vi "Capture.vi"(0 "Commands array":string[][](array[string])=[["Group20.825", "Group20.671", "Group20.814", "Group30.121"], ["Group2-0.528", "Group2-1.243", "Group2-0.539", "Group30.121"], ["Group20.374", "Group21.573", "Group20.363", "Group30.121"], ["Group2-0.242", "Group2-1.815", "Group2-0.253", "Group30.121"], ["Group20.165", "Group21.991", "Group20.154", "Group30.121"], ["Group2-0.077", "Group2-2.145", "Group2-0.088", "Group30.121"], ["Group20.044", "Group22.233", "Group20.033", "Group30.121"], ["Group2-2.310", "WT10", "WT10", "Group30.121"], ["Group22.310", "WT10", "WT10", "Group30.121"], ["Group2-2.310", "WT10", "WT10", "Group30.121"], ["Group22.310", "WT10", "WT10", "Group30.121"], ["Group2-2.310", "WT10", "WT10", "Group30.121"], ["Group22.310", "WT10", "WT10", "Group30.121"], ["Group2-0.011", "Group2-2.277", "Group2-0.022", "Group30.121"], ["Group20.066", "Group22.189", "Group20.055", "Group30.121"], ["Group2-0.121", "Group2-2.057", "Group2-0.132", "Group30.121"], ["Group20.209", "Group21.903", "Group20.198", "Group30.121"], ["Group2-0.297", "Group2-1.705", "Group2-0.308", "Group30.121"], ["Group20.451", "Group21.419", "Group20.440", "Group30.121"], ["Group2-0.660", "Group2-0.979", "Group2-0.671", "Group30.121"]], 1 "XPS_Address":string="192.168.254.254", 2 "VISA resource name":refnum<visa-resource-name>, 3 "laser array index":i32, 4 "Process time":dbl format="%#_13g", 5 "Axis Speed":dbl=1.0 format="%#_13g", 6 "Laser on/off array":bool[][](array[boolean])=[[FALSE, TRUE, FALSE, FALSE], [FALSE, TRUE, FALSE, FALSE], [FALSE, TRUE, FALSE, FALSE], [FALSE, TRUE, FALSE, FALSE], [FALSE, TRUE, FALSE, FALSE], [FALSE, TRUE, FALSE, FALSE], [FALSE, TRUE, FALSE, FALSE], [TRUE, FALSE, FALSE, FALSE], [TRUE, FALSE, FALSE, FALSE], [TRUE, FALSE, FALSE, FALSE], [TRUE, FALSE, FALSE, FALSE], [TRUE, FALSE, FALSE, FALSE], [TRUE, FALSE, FALSE, FALSE], [FALSE, TRUE, FALSE, FALSE], [FALSE, TRUE, FALSE, FALSE], [FALSE, TRUE, FALSE, FALSE], [FALSE, TRUE, FALSE, FALSE], [FALSE, TRUE, FALSE, FALSE], [FALSE, TRUE, FALSE, FALSE], [FALSE, TRUE, FALSE, FALSE]], 7 "stop":bool, 8 "delay before read (ms)":u32=500, 11 "Axis Initial Parameters":T1={"Velocity (units/seconds)"=1.0, "Acceleration (units/seconds²)"=20.0, "Minimum Jerk Time (seconds)"=0.005, "Maximum Jerk Time (seconds)"=0.009} {"Maximum Jerk Time (seconds)" format="%.6e"; "Minimum Jerk Time (seconds)" format="%.6e"; "Acceleration (units/seconds²)" format="%.6e"; "Velocity (units/seconds)" format="%.6e"}, 13 "ROI Area \n(mm2)":dbl=4.035870075999999, 14 "Axis 2":string="Group3", 15 "Axis 1":string="Group2", 17 "OPO on?":bool, 19 "Acceleration (units/seconds²)":dbl=20.0) -> (10 "Elapsed time":dbl, 16 "XPS error out":errorcluster, 18 "Error out":errorcluster)   [LabVIEW 2016]
uses:
  case selector.ctl
panel:
  out "Capture Log":string
  out "Axis 1 position":dbl format="%.10f"
  out "Axis 2 position":dbl format="%.10f"
  out "Initial time":timestamp
  in  "Active Positioner":string
  out "Current Line":i32
  out "1D Laser Array":bool[](array[boolean])=[FALSE, TRUE, FALSE, FALSE, FALSE, TRUE, FALSE, FALSE, FALSE, TRUE, FALSE, FALSE, FALSE, TRUE, FALSE, FALSE, FALSE, TRUE, FALSE, FALSE, FALSE, TRUE, FALSE, FALSE, FALSE, TRUE, FALSE, FALSE, TRUE, FALSE, FALSE, FALSE, TRUE, FALSE, FALSE, FALSE, TRUE, FALSE, FALSE, FALSE, TRUE, FALSE, FALSE, FALSE, TRUE, FALSE, FALSE, FALSE, TRUE, FALSE, FALSE, FALSE, FALSE, TRUE, FALSE, FALSE, FALSE, TRUE, FALSE, FALSE, FALSE, TRUE, FALSE, FALSE, FALSE, TRUE, FALSE, FALSE, FALSE, TRUE, FALSE, FALSE, FALSE, TRUE, FALSE, FALSE, FALSE, TRUE, FALSE, FALSE]
  out "1D command array":string[](array[string])=["Group20.825", "Group20.671", "Group20.814", "Group30.121", "Group2-0.528", "Group2-1.243", "Group2-0.539", "Group30.121", "Group20.374", "Group21.573", "Group20.363", "Group30.121", "Group2-0.242", "Group2-1.815", "Group2-0.253", "Group30.121", "Group20.165", "Group21.991", "Group20.154", "Group30.121", "Group2-0.077", "Group2-2.145", "Group2-0.088", "Group30.121", "Group20.044", "Group22.233", "Group20.033", "Group30.121", "Group2-2.310", "WT10", "WT10", "Group30.121", "Group22.310", "WT10", "WT10", "Group30.121", "Group2-2.310", "WT10", "WT10", "Group30.121", "Group22.310", "WT10", "WT10", "Group30.121", "Group2-2.310", "WT10", "WT10", "Group30.121", "Group22.310", "WT10", "WT10", "Group30.121", "Group2-0.011", "Group2-2.277", "Group2-0.022", "Group30.121", "Group20.066", "Group22.189", "Group20.055", "Group30.121", "Group2-0.121", "Group2-2.057", "Group2-0.132", "Group30.121", "Group20.209", "Group21.903", "Group20.198", "Group30.121", "Group2-0.297", "Group2-1.705", "Group2-0.308", "Group30.121", "Group20.451", "Group21.419", "Group20.440", "Group30.121", "Group2-0.660", "Group2-0.979", "Group2-0.671", "Group30.121"]
  out "Current Command":string
  out "Current laser element":bool
  out "Total lines":i32=80
  in  "Active Axis":string
  out "Laser on/off":bool
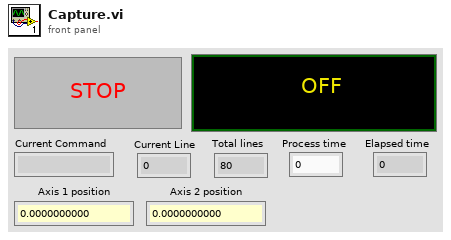
[diagram p1: front panel]
types:
  T1 = cluster{"Velocity (units/seconds)":dbl, "Acceleration (units/seconds²)":dbl, "Minimum Jerk Time (seconds)":dbl, "Maximum Jerk Time (seconds)":dbl}
  T2 = typedef "case selector.ctl" = enum16{"Initialize", "Element selection", "Laser", "Velocities", "Command", "Wait", "Exit"}
  T3 = enum16{"open", "replace", "create", "open or create", "replace or create", "replace or create with confirmation"}
  T4 = cluster{"connection TCP":refnum<k5>, "LogTo File":bool, "Log File refnum":refnum<file>, "no error if error log":bool}
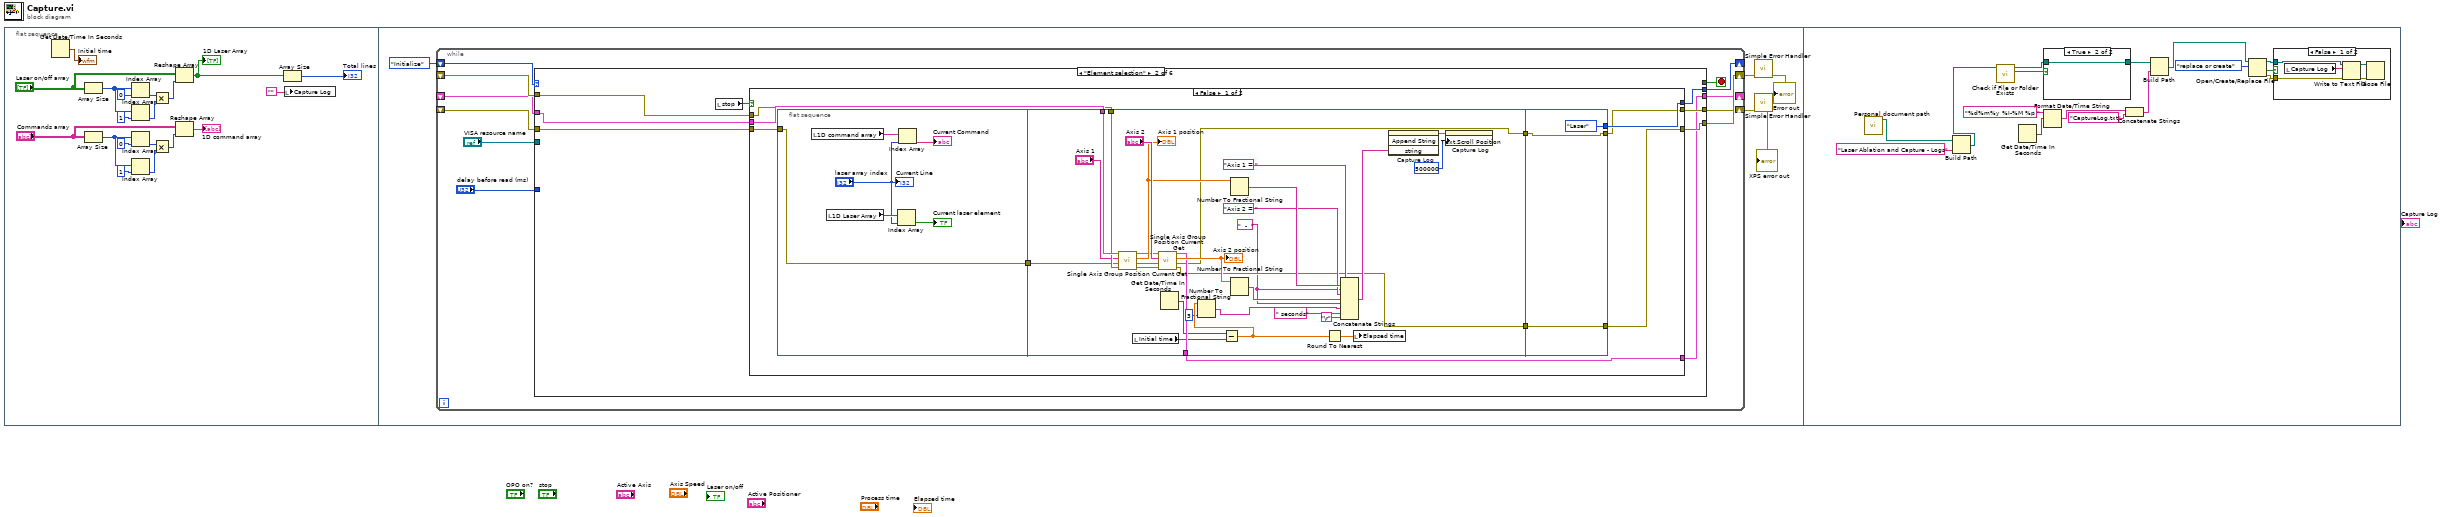
[diagram p0: block diagram]
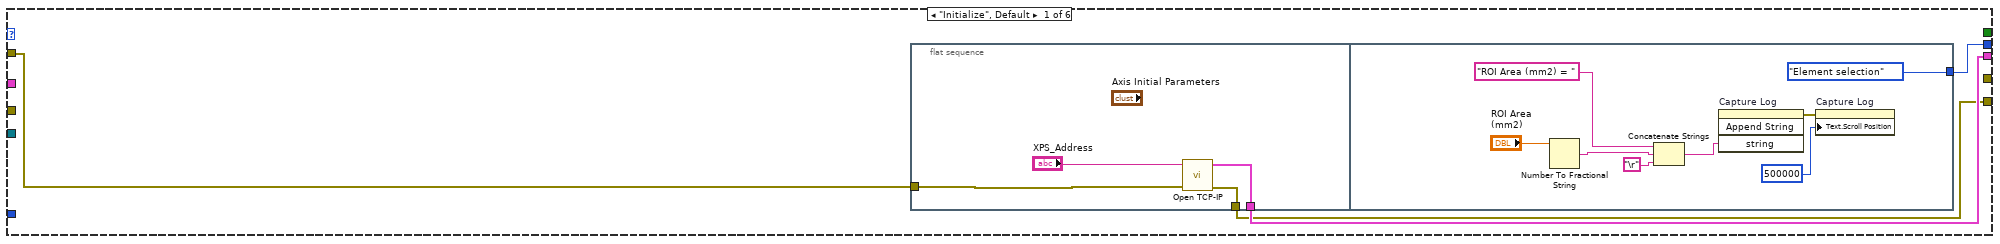
[diagram p2: hidden frame]
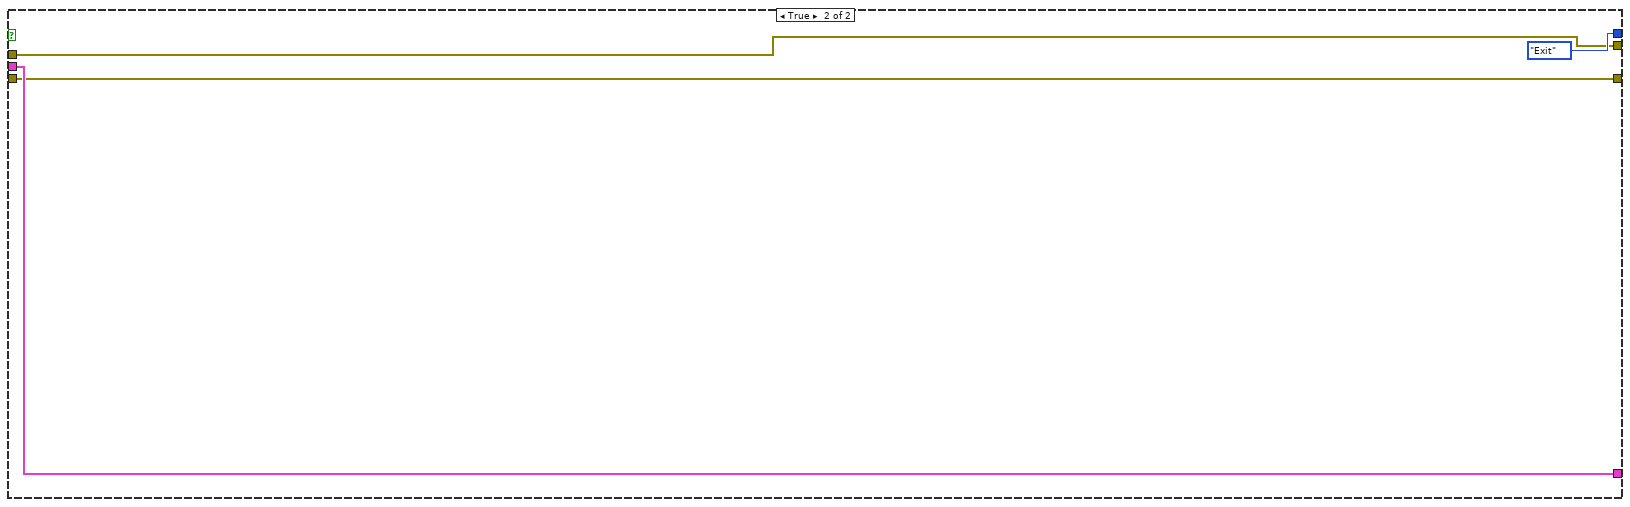
[diagram p3: hidden frame]
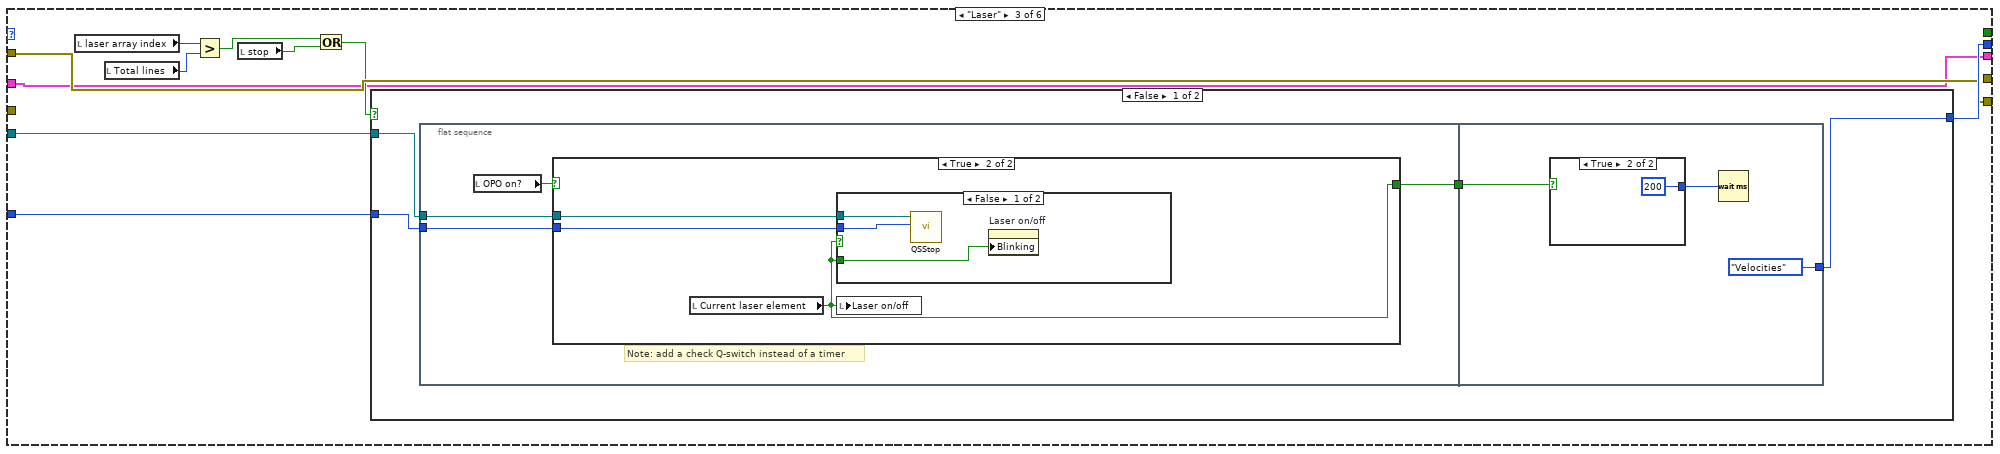
[diagram p4: hidden frame]
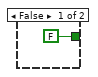
[diagram p5: hidden frame]
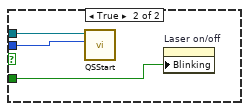
[diagram p6: hidden frame]
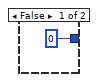
[diagram p7: hidden frame]
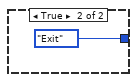
[diagram p8: hidden frame]
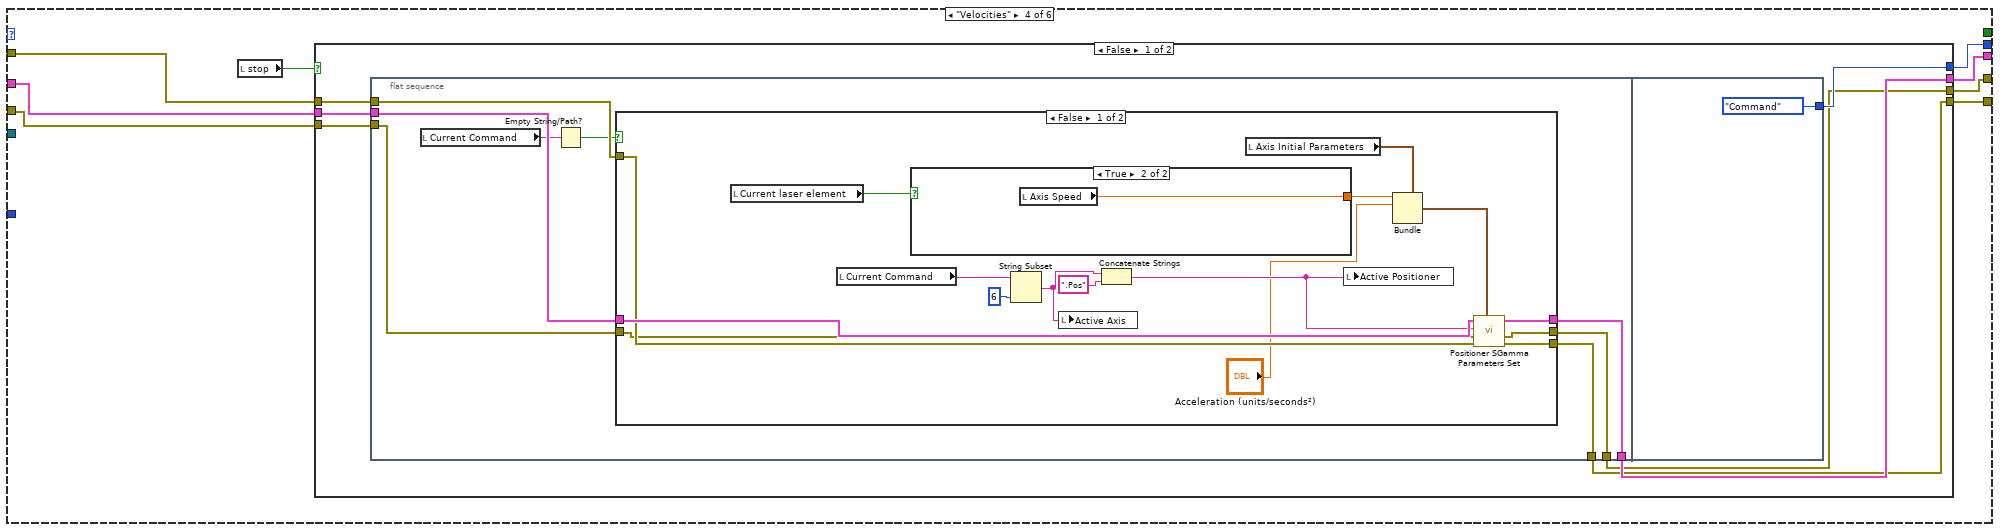
[diagram p9: hidden frame]
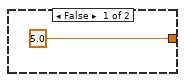
[diagram p10: hidden frame]
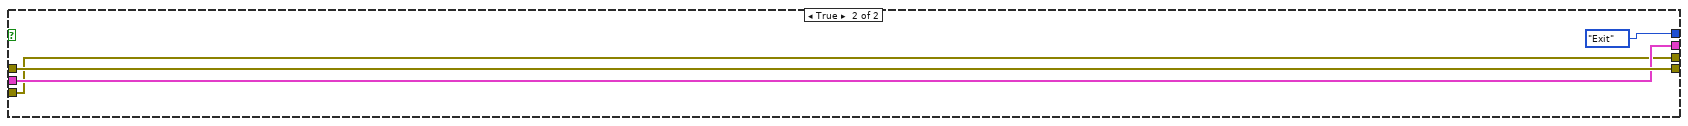
[diagram p12: hidden frame]
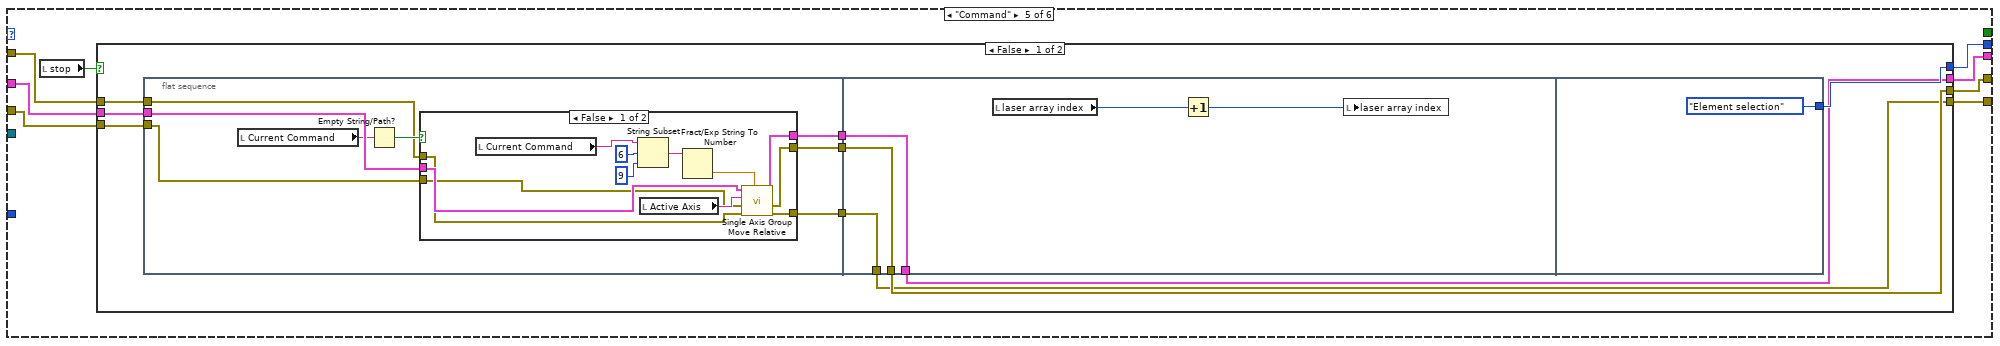
[diagram p13: hidden frame]
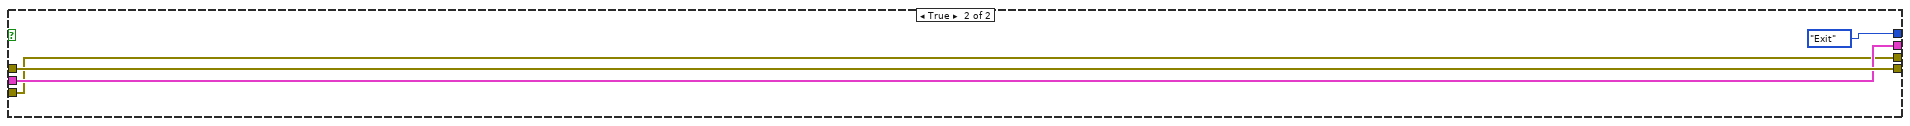
[diagram p15: hidden frame]
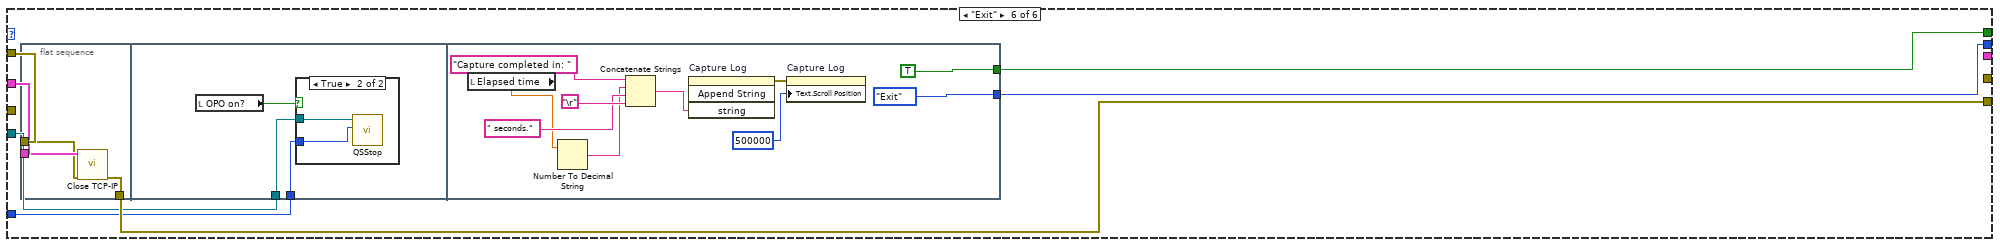
[diagram p16: hidden frame]
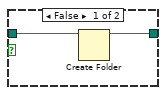
[diagram p18: hidden frame]
diagram:
  n1 = flat-sequence {
    frame #0 {
      n2 = Get Date/Time In Seconds() -> (seconds since 1Jan1904=→"Initial time":timestamp)
      n3 = Array Size(array="Commands array") -> (size(s)=w3:i32[])
      n4 = Array Size(array="Laser on/off array") -> (size(s)=w11:i32[])
      n5 = Index Array(array=w11, index=0) -> (element=w14:i32)
      n6 = Index Array(array=w11, index=1) -> (element=w15:i32)
      n7 = Index Array(array=w3, index=0) -> (element=w6:i32)
      n8 = Index Array(array=w3, index=1) -> (element=w7:i32)
      n9 = Multiply(x=w14, y=w15) -> (x*y=w16:i32)
      n10 = Multiply(x=w6, y=w7) -> (x*y=w8:i32)
      n11 = Reshape Array("Laser on/off array", w16) -> (w19:bool[])
      "1D Laser Array" <- w19
      n12 = Reshape Array("Commands array", w8) -> (→"1D command array":string[])
      n13 = Array Size(array=w19) -> (size(s)=→"Total lines":i32)
      n14 = local write "Capture Log"("") -> ()
    }
    frame #1 {
      n15 = while {
        shift-right: [w32] -> _
        shift-left: case_selector."Initialize" -> [w33]
        shift-right: [w30] -> w20
        shift-left: _ -> [w31]
        shift-right: [w29] -> _
        shift-left: _ -> [w28]
        shift-right: [w27] -> w21
        shift-left: _ -> [w26]
        stop <- w25 stop-if-true
        n16 = case shown="\"Element selection\"" w33 {
          tunnel: [w37 w57 w119 w151 w200 w247] -> w32
          tunnel: w31 -> [w36 w54 w118 w149 w198 w248]
          tunnel: [w34 w51 w118 w148 w197 w246] -> w30
          tunnel: [w35 w50 w112 w146 w195 _] -> w29
          tunnel: w28 -> [_ w55 w112 w147 w196 w245]
          tunnel: [_ w52 _ w145 w193 _] -> w27
          tunnel: w26 -> [_ w53 _ w144 w194 _]
          tunnel: [_ _ _ _ _ w244] -> w25
          tunnel: "VISA resource name" -> [_ _ w111 _ _ w242]
          tunnel: "delay before read (ms)" -> [_ _ w110 _ _ w243]
          frame "Initialize", Default {
            n17 = flat-sequence {
              tunnel: w36 -> [w40]
              tunnel: [w39] -> w35
              tunnel: [w38] -> w34
              tunnel: [case_selector."Element selection"] -> w37
              frame #0 {
                n18 = call <userlib>:"Open TCP-IP.vi"("error in (no error)"=w40, "IP address"="XPS_Address") -> ("error out"=w38:errorcluster, "Connection ID"=w39:T4)  [unwired: 7 in, 1 out]
              }
              frame #1 {
                n19 = Number To Fractional String(number="ROI Area \n(mm2)") -> (F-format string=w45:string)  [unwired: 3 in]
                n20 = Concatenate Strings("ROI Area (mm2) = " ("string"), w45, "\r") -> (w43:string)
                n21 = invoke on="Capture Log" class="Str" method="Append String"("string"=w43) -> (error out=w47:errorcluster)  [unwired: 3 in, 3 out]
                n22 = property on="Capture Log" class="Str"(error in=w47, "Text.Scroll Position"=u32 500000) -> ()  [unwired: 1 in, 2 out]
              }
            }
          }
          frame "Element selection" {
            n23 = local read "stop"() -> (w56:bool)
            n24 = case shown="False" w56 {
              tunnel: [w66 case_selector."Exit"] -> w57
              tunnel: w55 -> [w67 w108]
              tunnel: w54 -> [w60 w107]
              tunnel: w53 -> [w59 w106]
              tunnel: [w61 w107] -> w52
              tunnel: [w63 w106] -> w51
              tunnel: [w65 w108] -> w50
              frame False {
                n25 = flat-sequence {
                  tunnel: w59 -> [w68]
                  tunnel: [w68] -> w58
                  tunnel: w67 -> [w95]
                  tunnel: w60 -> [w93]
                  tunnel: [w86] -> w65
                  tunnel: [w85] -> w64
                  tunnel: [w84] -> w62
                  tunnel: w58 -> [w83]
                  tunnel: [case_selector."Laser"] -> w66
                  tunnel: w64 -> [w104]
                  tunnel: [w104] -> w63
                  tunnel: w62 -> [w103]
                  tunnel: [w103] -> w61
                  frame #0 {
                    n26 = local read "1D command array"() -> (w71:string[])
                    n27 = local read "1D Laser Array"() -> (w70:bool[])
                    n28 = Index Array(array=w70, index="laser array index") -> (element=→"Current laser element":bool)
                    n29 = Index Array(array=w71, index="laser array index") -> (element=→"Current Command":string)
                    "Current Line" <- "laser array index"
                  }
                  frame #1 {
                    w82 = "  -  " ("string")
                    n30 = call <userlib>:"Single Axis Group Position Current Get.vi"("error in (no error)"=w93, "XPS error in (no error)"=w83, "SingleAxis Group  Name (250 c max)"="Axis 1", "connection ID in"=w95) -> ("error out"=w87:errorcluster, "XPS error out"=w88:errorcluster, "Current Position (units)"=w92:dbl, "connection ID out"=w89:T4)  [unwired: 4 in]
                    "Axis 1 position" <- w92
                    n31 = local read "Initial time"() -> (w79:timestamp)
                    n32 = call <userlib>:"Single Axis Group Position Current Get.vi"("error in (no error)"=w87, "XPS error in (no error)"=w88, "SingleAxis Group  Name (250 c max)"="Axis 2", "connection ID in"=w89) -> ("error out"=w85:errorcluster, "XPS error out"=w84:errorcluster, "Current Position (units)"=w91:dbl, "connection ID out"=w86:T4)  [unwired: 4 in]
                    "Axis 2 position" <- w91
                    n33 = Get Date/Time In Seconds() -> (seconds since 1Jan1904=w80:timestamp)
                    n34 = Subtract(x=w80, y=w79) -> (x-y=w75:dbl)
                    n35 = Number To Fractional String(number=w75, precision (6)=i16 3) -> (F-format string=w78:string)  [unwired: 2 in]
                    n36 = Number To Fractional String(number=w92) -> (F-format string=w101:string)  [unwired: 3 in]
                    n37 = Number To Fractional String(number=w91) -> (F-format string=w100:string)  [unwired: 3 in]
                    n38 = Round To Nearest(number=w75) -> (nearest integer value=w81:dbl)
                    n39 = Concatenate Strings("Axis 1 = " ("string"), w101, w82, "Axis 2 = " ("string"), w100, w82, w78, " seconds" ("milliseconds"), "\r") -> (w98:string)
                    n40 = local write "Elapsed time"(w81) -> ()
                    n41 = invoke on="Capture Log" class="Str" method="Append String"("string"=w98) -> (error out=w97:errorcluster)  [unwired: 3 in, 3 out]
                    n42 = property on="Capture Log" class="Str"(error in=w97, "Text.Scroll Position"=u32 500000) -> ()  [unwired: 1 in, 2 out]
                  }
                  frame #2 {
                  }
                }
              }
              frame True {
              }
            }
          }
          frame "Laser" {
            n43 = local read "laser array index"() -> (w116:i32)
            n44 = local read "Total lines"() -> (w117:i32)
            n45 = Greater?(x=w116, y=w117) -> (0:w114:bool)
            n46 = local read "stop"() -> (w115:bool)
            n47 = Or(x=w114, y=w115) -> (x .or. y?=w113:bool)
            n48 = case shown="False" w113 {
              tunnel: [w123 case_selector."Exit"] -> w119
              tunnel: w111 -> [w121 _]
              tunnel: w110 -> [w120 _]
              frame False {
                n49 = flat-sequence {
                  tunnel: [w126] -> w122
                  tunnel: w121 -> [w125]
                  tunnel: w120 -> [w124]
                  tunnel: [case_selector."Velocities"] -> w123
                  tunnel: w122 -> [w139]
                  frame #0 {
                    # "Note: add a check Q-switch instead of a timer"
                    n50 = local read "OPO on?"() -> (w127:bool)
                    n51 = case shown="True" w127 {
                      tunnel: [FALSE ("Current laser element") w131] -> w126
                      tunnel: w125 -> [_ w130]
                      tunnel: w124 -> [_ w129]
                      frame False {
                      }
                      frame True {
                        n52 = local read "Current laser element"() -> (w131:bool)
                        n53 = case shown="False" w131 {
                          tunnel: w131 -> [w134 w137]
                          tunnel: w130 -> [w133 w136]
                          tunnel: w129 -> [w132 w135]
                          frame False {
                            n54 = call "QSStop.vi"("delay before read (ms)"=w132, "VISA resource name"=w133) -> ()  [unwired: 6 in, 4 out]
                            n55 = property on="Laser on/off" class="Bool (strict)"("Blinking"=w134) -> ()  [unwired: 2 in, 2 out]
                          }
                          frame True {
                            n56 = call "QSStart.vi"("delay before read (ms)"=w135, "VISA resource name"=w136) -> ()  [unwired: 6 in, 4 out]
                            n57 = property on="Laser on/off" class="Bool (strict)"("Blinking"=w137) -> ()  [unwired: 2 in, 2 out]
                          }
                        }
                        n58 = local write "Laser on/off"(w131) -> ()
                      }
                    }
                  }
                  frame #1 {
                    n59 = case shown="True" w139 {
                      tunnel: [u32 0 ("milliseconds to wait") u32 200 ("milliseconds to wait")] -> w138
                      frame False {
                      }
                      frame True {
                      }
                    }
                    n60 = Wait (ms)(milliseconds to wait=w138) -> ()  [unwired: 1 out]
                  }
                }
              }
              frame True {
              }
            }
          }
          frame "Velocities" {
            n61 = local read "stop"() -> (w150:bool)
            n62 = case shown="False" w150 {
              tunnel: [w158 case_selector."Exit"] -> w151
              tunnel: w149 -> [w157 w191]
              tunnel: [w154 w191] -> w148
              tunnel: w147 -> [w156 w190]
              tunnel: [w155 w190] -> w146
              tunnel: [w153 w189] -> w145
              tunnel: w144 -> [w152 w189]
              frame False {
                n63 = flat-sequence {
                  tunnel: w157 -> [w164]
                  tunnel: w156 -> [w166]
                  tunnel: [w165] -> w155
                  tunnel: [w163] -> w154
                  tunnel: [w162] -> w153
                  tunnel: w152 -> [w161]
                  tunnel: [case_selector."Command"] -> w158
                  frame #0 {
                    n64 = local read "Current Command"() -> (w160:string)
                    n65 = Empty String/Path?(string/path=w160) -> (empty?=w159:bool)
                    n66 = case shown="False" w159 {
                      tunnel: w166 -> [w179 w185]
                      tunnel: [w178 w185] -> w165
                      tunnel: w164 -> [w177 w186]
                      tunnel: [w176 w186] -> w163
                      tunnel: [w171 w187] -> w162
                      tunnel: w161 -> [w170 w187]
                      frame False {
                        n67 = local read "Current laser element"() -> (w182:bool)
                        n68 = local read "Current Command"() -> (w180:string)
                        n69 = case shown="True" w182 {
                          tunnel: [5.0 w184] -> w175
                          frame False {
                          }
                          frame True {
                            n70 = local read "Axis Speed"() -> (w184:dbl)
                          }
                        }
                        n71 = String Subset(string=w180, length (rest)=6 ("length (rest)")) -> (substring=w169:string)  [unwired: 1 in]
                        n72 = local write "Active Axis"(w169) -> ()
                        n73 = Concatenate Strings(w169, ".Pos" ("string")) -> (w168:string)
                        n74 = local read "Axis Initial Parameters"() -> (w173:T1)
                        n75 = local write "Active Positioner"(w168) -> ()
                        n76 = Bundle(cluster=w173, "Velocity (units/seconds)"=w175, "Acceleration (units/seconds²)"="Acceleration (units/seconds²)") -> (w174:T1)  [unwired: 2 in]
                        n77 = call <userlib>:"Positioner SGamma Parameters Set.vi"("SGamma Parameters"=w174, "error in (no error)"=w177, "XPS error in (no error)"=w170, "Positioner Name (250 c max)"=w168, "connection ID in"=w179) -> ("error out"=w176:errorcluster, "XPS error out"=w171:errorcluster, "connection ID out"=w178:T4)  [unwired: 4 in]
                      }
                      frame True {
                      }
                    }
                  }
                  frame #1 {
                  }
                }
              }
              frame True {
              }
            }
          }
          frame "Command" {
            n78 = local read "stop"() -> (w199:bool)
            n79 = case shown="False" w199 {
              tunnel: [w204 case_selector."Exit"] -> w200
              tunnel: w198 -> [w208 w240]
              tunnel: [w202 w240] -> w197
              tunnel: w196 -> [w210 w239]
              tunnel: [w201 w239] -> w195
              tunnel: w194 -> [w207 w238]
              tunnel: [w203 w238] -> w193
              frame False {
                n80 = flat-sequence {
                  tunnel: w210 -> [w218]
                  tunnel: [w217] -> w209
                  tunnel: w208 -> [w214]
                  tunnel: w207 -> [w213]
                  tunnel: [w212] -> w206
                  tunnel: [w211] -> w205
                  tunnel: w209 -> [w232]
                  tunnel: w206 -> [w234]
                  tunnel: w205 -> [w233]
                  tunnel: [w234] -> w203
                  tunnel: [w233] -> w202
                  tunnel: [w232] -> w201
                  tunnel: [case_selector."Element selection"] -> w204
                  frame #0 {
                    n81 = local read "Current Command"() -> (w215:string)
                    n82 = Empty String/Path?(string/path=w215) -> (empty?=w216:bool)
                    n83 = case shown="False" w216 {
                      tunnel: w218 -> [w230 w231]
                      tunnel: [w223 w231] -> w217
                      tunnel: w214 -> [w222 _]
                      tunnel: w213 -> [w221 _]
                      tunnel: [w220 _] -> w212
                      tunnel: [w219 _] -> w211
                      frame False {
                        n84 = local read "Current Command"() -> (w229:string)
                        n85 = String Subset(string=w229, offset (0)=6, length (rest)=9 ("length (rest)")) -> (substring=w226:string)
                        n86 = local read "Active Axis"() -> (w224:string)
                        n87 = Fract/Exp String To Number(string=w226) -> (number=w225:dbl)  [unwired: 3 in, 1 out]
                        n88 = call <userlib>:"Single Axis Group Move Relative.vi"("Target Displacement (units)"=w225, "error in (no error)"=w222, "XPS error in (no error)"=w221, "SingleAxis Group  Name (250 c max)"=w224, "connection ID in"=w230) -> ("error out"=w219:errorcluster, "XPS error out"=w220:errorcluster, "connection ID out"=w223:T4)  [unwired: 4 in]
                      }
                      frame True {
                      }
                    }
                  }
                  frame #1 {
                    n89 = local read "laser array index"() -> (w236:i32)
                    n90 = Increment(x=w236) -> (x+1=w235:i32)
                    n91 = local write "laser array index"(w235) -> ()
                  }
                  frame #2 {
                  }
                }
              }
              frame True {
              }
            }
          }
          frame "Exit" {
            n92 = flat-sequence {
              tunnel: w248 -> [w250]
              tunnel: [w249] -> w246
              tunnel: w245 -> [w251]
              tunnel: w243 -> [w253]
              tunnel: w242 -> [w252]
              tunnel: [case_selector."Exit"] -> w247
              tunnel: [TRUE] -> w244
              frame #0 {
                n93 = call <userlib>:"Close TCP-IP.vi"("error in (no error)"=w250, "connection ID in"=w251) -> ("Error out"=w249:errorcluster)  [unwired: 9 in]
              }
              frame #1 {
                n94 = local read "OPO on?"() -> (w254:bool)
                n95 = case shown="True" w254 {
                  tunnel: w253 -> [_ w256]
                  tunnel: w252 -> [_ w255]
                  frame False {
                  }
                  frame True {
                    n96 = call "QSStop.vi"("delay before read (ms)"=w256, "VISA resource name"=w255) -> ()  [unwired: 6 in, 4 out]
                  }
                }
              }
              frame #2 {
                n97 = local read "Elapsed time"() -> (w258:dbl)
                n98 = Number To Decimal String(number=w258) -> (decimal integer string=w257:string)  [unwired: 1 in]
                n99 = Concatenate Strings("Capture completed in: " ("string"), w257, " seconds." ("string"), "\r") -> (w259:string)
                n100 = invoke on="Capture Log" class="Str" method="Append String"("string"=w259) -> (error out=w264:errorcluster)  [unwired: 3 in, 3 out]
                n101 = property on="Capture Log" class="Str"(error in=w264, "Text.Scroll Position"=u32 500000) -> ()  [unwired: 1 in, 2 out]
              }
            }
          }
        }
      }
      "XPS error out" <- w21
      "Error out" <- w20
      n102 = call <vilib>:"Simple Error Handler.vi"("error in (no error)"=w20) -> ()  [unwired: 4 in, 5 out]
      n103 = call <vilib>:"Simple Error Handler.vi"("error in (no error)"=w21) -> ()  [unwired: 4 in, 5 out]
    }
    frame #2 {
      n104 = call "Personal document path.vi"() -> ("My Documents"=w268:path)  [unwired: 10 in, 1 out]
      n105 = Build Path(base path=w268, name or relative path="Laser Ablation and Capture - Logs") -> (appended path=w267:path)
      n106 = call <vilib>:"Check if File or Folder Exists.vi"("path"=w267) -> ("file or folder exists?"=w277:bool, "dup path"=w276:path)  [unwired: 8 in, 1 out]
      n107 = Get Date/Time In Seconds() -> (seconds since 1Jan1904=w279:timestamp)
      n108 = case shown="True" w277 {
        tunnel: w276 -> [w284 w285]
        tunnel: [w283 w285] -> w273
        frame False {
          n109 = Create Folder(path (use dialog)=w284) -> (created path=w283:path)  [unwired: 2 in, 2 out]
        }
        frame True {
        }
      }
      n110 = Format Date/Time String(time format string (%c)="%d%m%y %I-%M %p ", seconds (now)=w279) -> (date/time string=w281:string)  [unwired: 1 in]
      n111 = Concatenate Strings(w281, "CaptureLog.txt") -> (w274:string)
      n112 = Build Path(base path=w273, name or relative path=w274) -> (appended path=w275:path)
      n113 = Open/Create/Replace File(file path (use dialog)=w275, operation (0:open)=T3."replace or create") -> (refnum out=w272:refnum<file>, cancelled=w270:bool, error out=w271:errorcluster)  [unwired: 4 in]
      n114 = case shown="False" w270 {
        tunnel: w272 -> [w290 _]
        tunnel: w271 -> [w288 _]
        frame False {
          n115 = local read "Capture Log"() -> (w289:string)
          n116 = Write to Text File(file (use dialog)=w290, text=w289, error in=w288) -> (refnum out=w287:refnum<file>, error out=w286:errorcluster)  [unwired: 2 out]
          n117 = Close File(refnum=w287, error in=w286) -> ()  [unwired: 2 out]
        }
        frame True {
        }
      }
    }
  }
